vi "IZRCSM_ut_test_eng.vi"(8 "Error In":errorcluster, 11 "CSMinfo in":T2) -> (0 "Error Out":errorcluster, 3 "CSMinfo out":T2)   [LabVIEW 2018]
uses:
  IZRCSM.ctl
  IZRCSM_string2.ctl
  MOKO_LabViewLibrary/MokoSTM/MokoClassicUtilitySTM/MCUS_STM.ctl
  MOKO_LabViewLibrary/MokoSTM/MokoClassicUtilitySTM/MCUS_ITEM.ctl
panel:
  in  "Применить":bool
  in  "Температура окружающего воздуха":T1
  in  "Атмосферное давление":T1
  in  "Относительная влажность воздуха":T1
  # "0,4\n0,6\n1\n1,5\n1,6\n2,5\n4"
  # "kPa\nbar\nkgf/cm2\nMPa"
  # "Climatic conditions"
  # "Permissible range"
  # "Measured values"
  # "Measured parameter"
  # "Ambient temperature:"
  # "from +15,0 °C to +35,0 °C"
  # "Relative humidity:"
  # "from 45% to 80%"
  # "Atmosphere pressure:"
  # "from 84,0 to 106,7 kPa"
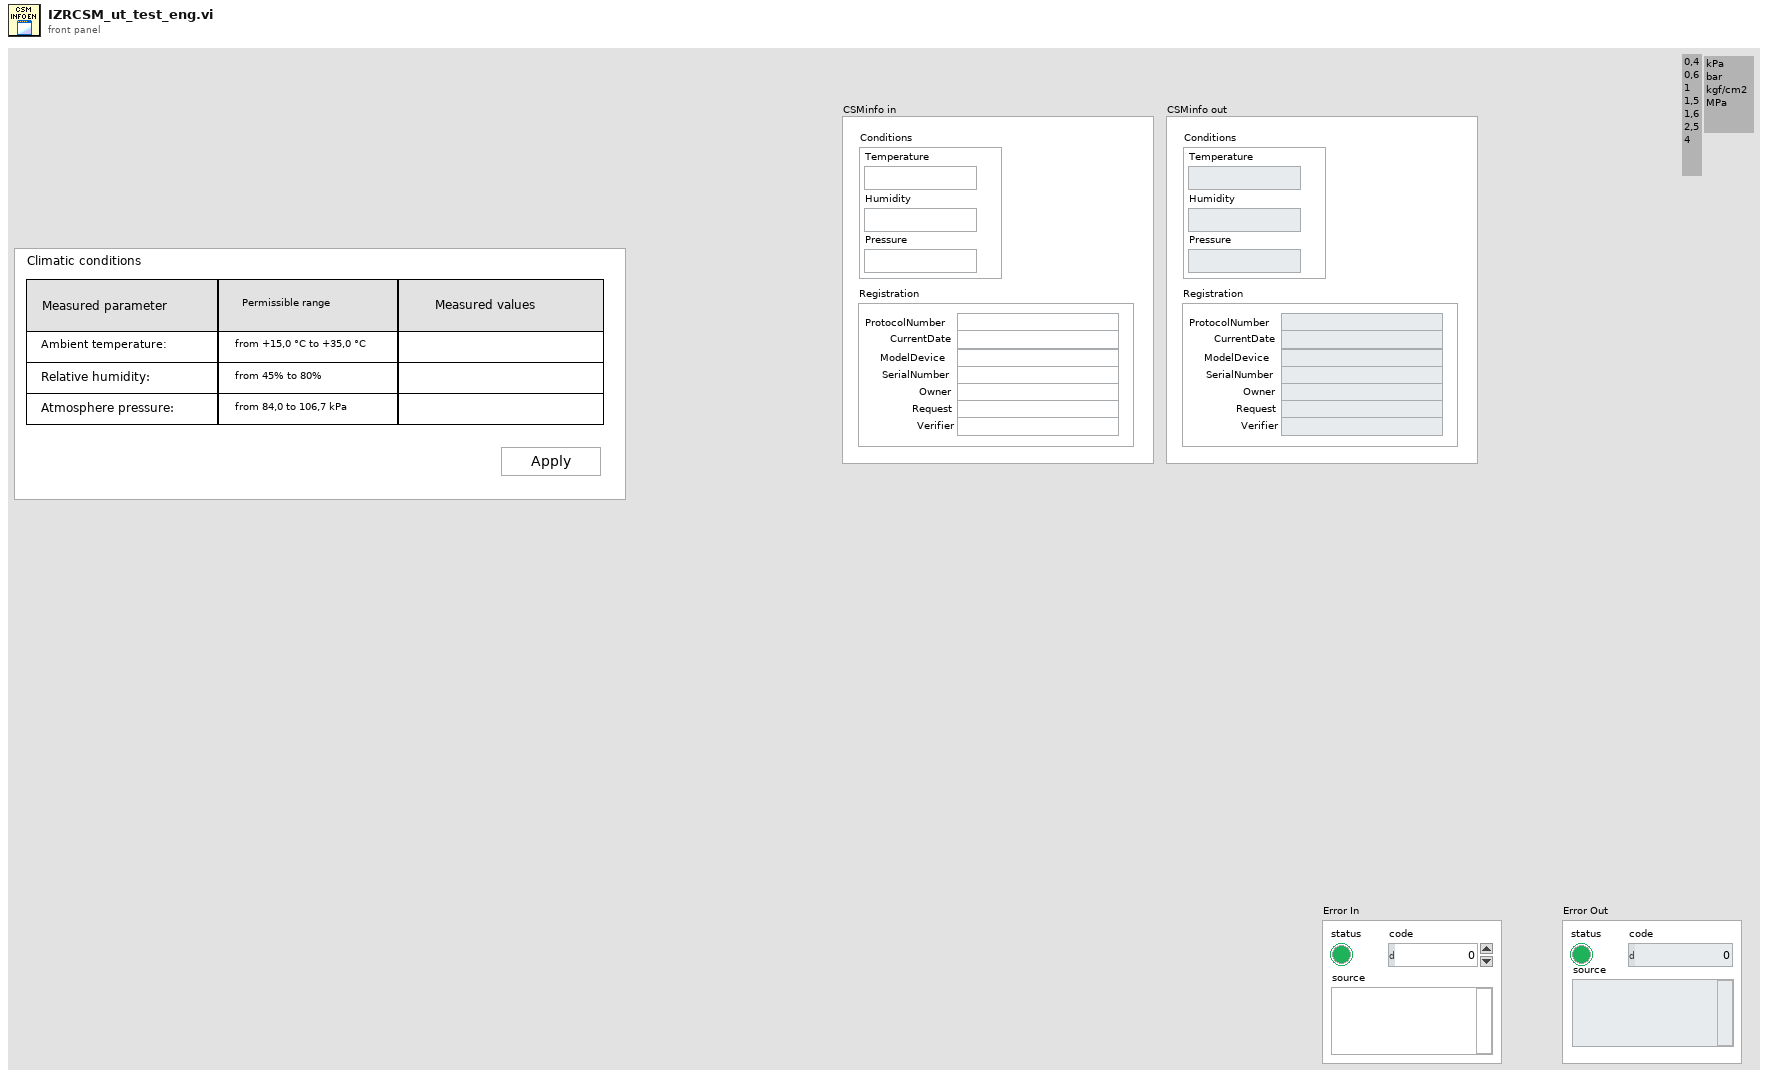
[diagram p1: front panel]
types:
  T1 = typedef "IZRCSM_string2.ctl" = string
  T2 = typedef "IZRCSM.ctl" = cluster{"Conditions":cluster{"Temperature":string, "Humidity":string, "Pressure":string}, "Registration":cluster{"ProtocolNumber":string, "CurrentDate":string, "ModelDevice":string, "SerialNumber":string, "Owner":string, "Request":string, "Verifier":string}}
  T3 = typedef "MCUS_STM.ctl" = cluster{"main stm":T4, "data":string}
  T4 = typedef "MCUS_ITEM.ctl" = enum16{"idle", "_____ main_____ ", "Init", "Stop", "Apply values", "Save", "Open", "Reset"}
  T5 = typedef "CSMinfo_string2.ctl" = string
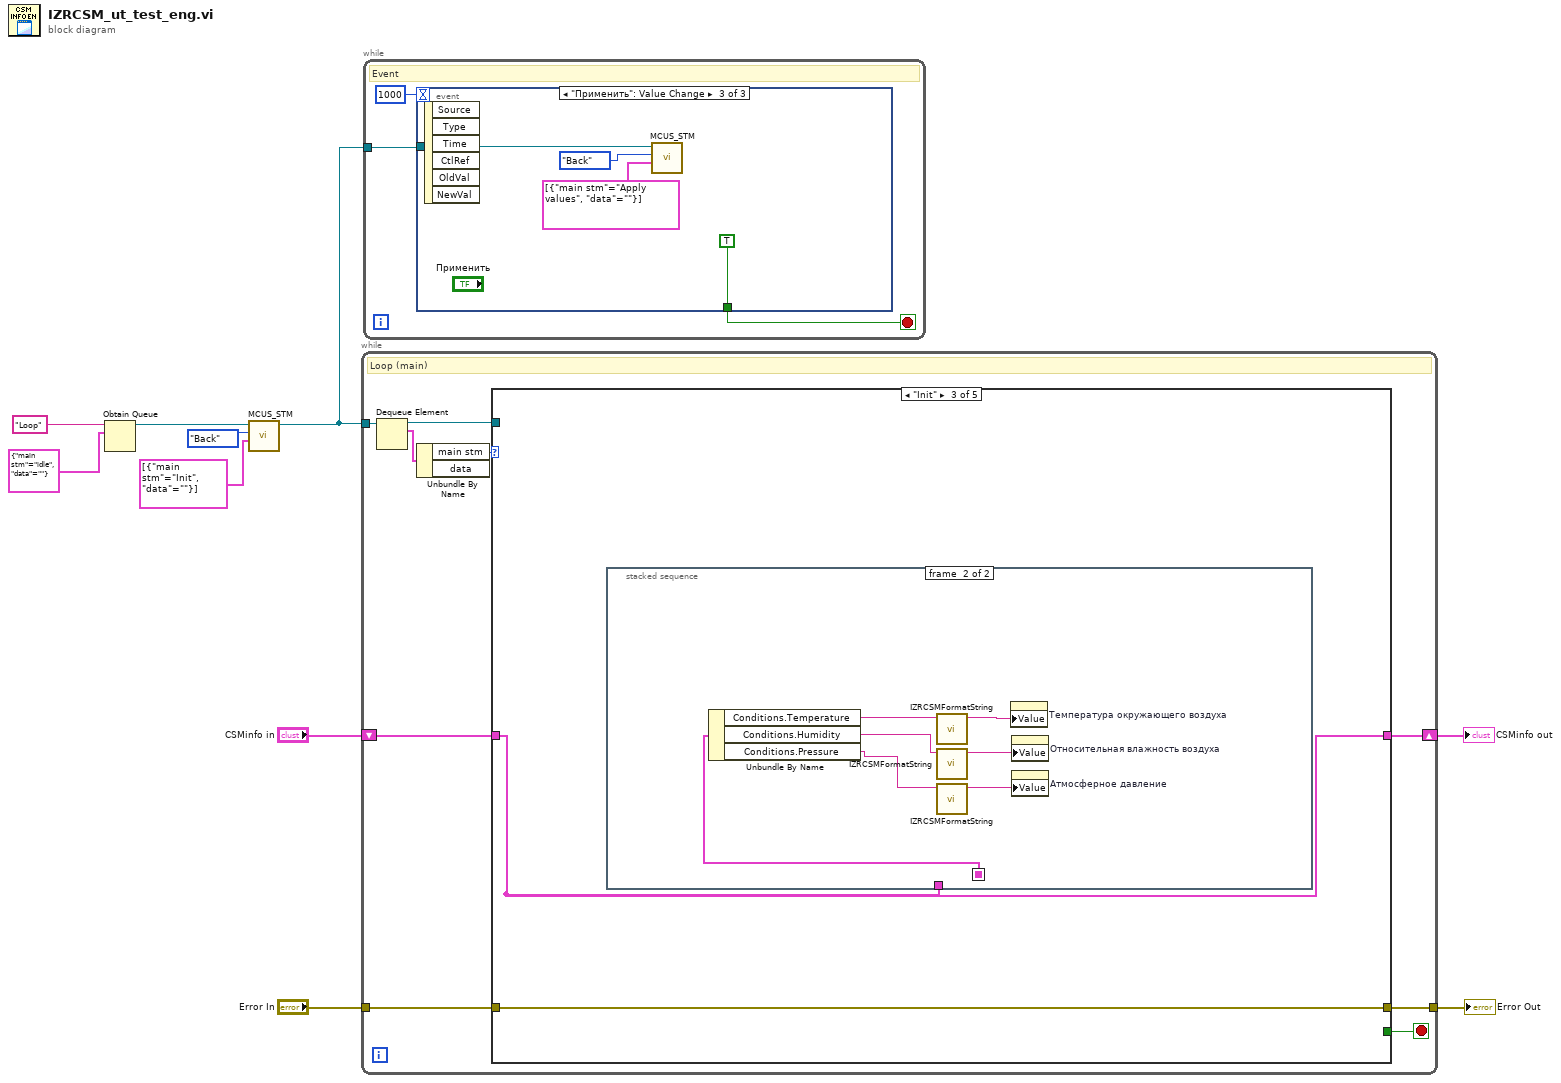
[diagram p0: block diagram]
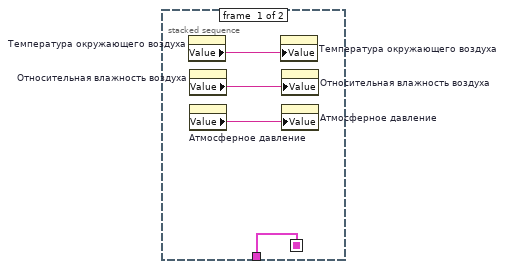
[diagram p4: hidden frame]
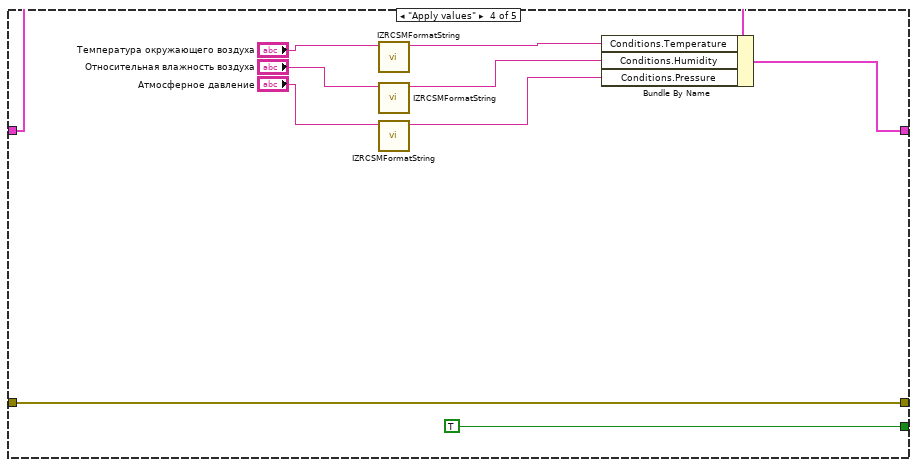
[diagram p5: hidden frame]
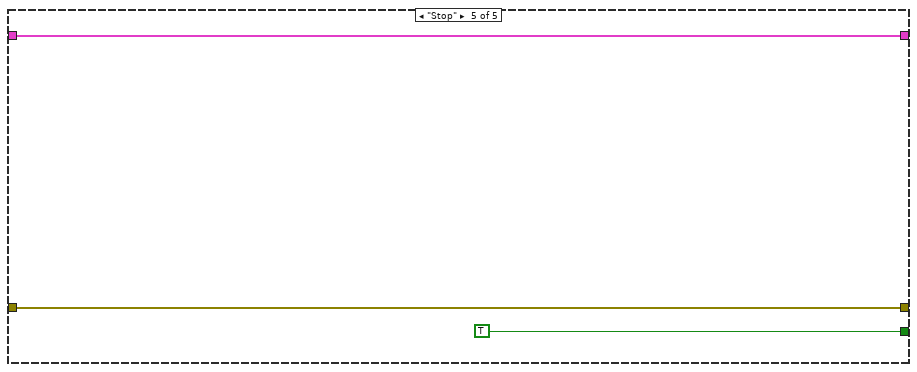
[diagram p6: hidden frame]
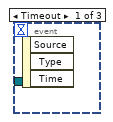
[diagram p7: hidden frame]
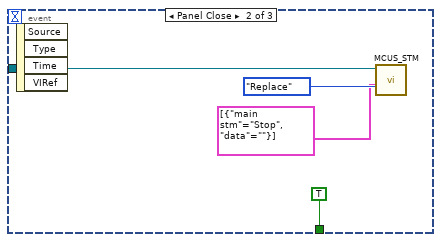
[diagram p8: hidden frame]
diagram:
  n1 = Obtain Queue(name (unnamed)="Loop", element data type=T3 {"main stm"=enum."idle", "data"=""} ("MOKO_NMEA")) -> (queue out=w10:refnum<queue>)  [unwired: 3 in, 2 out]
  n2 = call "MCUS_STM.vi"("StateMachineSteps"=T3[] [{"main stm"=enum."Init", "data"=""}], "FNs"=enum16{"Back", "Front", "Replace"}."Back", "Queue in"=w10) -> ("Queue out"=w5:refnum<queue>)  [unwired: 7 in, 1 out]
  n3 = while {
    tunnel: w5 -> [w19]
    tunnel: "Error In" -> [w12]
    tunnel: [w11] -> w1
    shift-right: [w14] -> w4
    shift-left: "CSMinfo in" -> [w13]
    stop <- w15 stop-if-true
    # "Loop (main)"
    n4 = Dequeue Element(queue=w19) -> (queue out=w18:refnum<queue>, element=w17:T3)  [unwired: 2 in, 2 out]
    n5 = Unbundle By Name(w17) -> ("main stm"=w16:T4)  [unwired: 1 out]
    n6 = case shown="\"Init\"" w16 {
      tunnel: w18 -> [_ _ _ _ _]
      tunnel: [_ _ _ TRUE TRUE] -> w15
      tunnel: [_ _ w20 w36 w44] -> w14
      tunnel: w13 -> [_ _ w20 w37 w44]
      tunnel: w12 -> [_ _ w21 w41 w43]
      tunnel: [_ _ w21 w41 w43] -> w11
      frame "idle", Default {
      }
      frame "_____ main_____ " {
      }
      frame "Init" {
        n7 = stacked-sequence {
          seq-local: [w25 _] -> [_ w26]
          tunnel: w20 -> [w25 _]
          frame #0 {
            n8 = property on="Температура окружающего воздуха" class="Str (strict)"() -> ("Value"=w24:T5)  [unwired: 2 in, 2 out]
            n9 = property on="Относительная влажность воздуха" class="Str (strict)"() -> ("Value"=w23:T5)  [unwired: 2 in, 2 out]
            n10 = property on="Атмосферное давление" class="Str (strict)"() -> ("Value"=w22:T5)  [unwired: 2 in, 2 out]
            n11 = property on="Температура окружающего воздуха" class="Str (strict)"("Value"=w24) -> ()  [unwired: 2 in, 2 out]
            n12 = property on="Относительная влажность воздуха" class="Str (strict)"("Value"=w23) -> ()  [unwired: 2 in, 2 out]
            n13 = property on="Атмосферное давление" class="Str (strict)"("Value"=w22) -> ()  [unwired: 2 in, 2 out]
          }
          frame #1 {
            n14 = Unbundle By Name(w26) -> ("Conditions.Temperature"=w29:string, "Conditions.Humidity"=w28:string, "Conditions.Pressure"=w27:string)
            n15 = call "IZRCSMFormatString.vi"("Input string"=w29) -> ("resulting string"=w31:string)  [unwired: 9 in, 1 out]
            n16 = call "IZRCSMFormatString.vi"("Input string"=w28) -> ("resulting string"=w30:string)  [unwired: 9 in, 1 out]
            n17 = call "IZRCSMFormatString.vi"("Input string"=w27) -> ("resulting string"=w32:string)  [unwired: 9 in, 1 out]
            n18 = property on="Температура окружающего воздуха" class="Str (strict)"("Value"=w31) -> ()  [unwired: 2 in, 2 out]
            n19 = property on="Относительная влажность воздуха" class="Str (strict)"("Value"=w30) -> ()  [unwired: 2 in, 2 out]
            n20 = property on="Атмосферное давление" class="Str (strict)"("Value"=w32) -> ()  [unwired: 2 in, 2 out]
          }
        }
      }
      frame "Apply values" {
        n21 = call "IZRCSMFormatString.vi"("Input string"="Температура окружающего воздуха") -> ("resulting string"=w35:string)  [unwired: 9 in, 1 out]
        n22 = call "IZRCSMFormatString.vi"("Input string"="Относительная влажность воздуха") -> ("resulting string"=w34:string)  [unwired: 9 in, 1 out]
        n23 = call "IZRCSMFormatString.vi"("Input string"="Атмосферное давление") -> ("resulting string"=w33:string)  [unwired: 9 in, 1 out]
        n24 = Bundle By Name(cluster=w37, "Conditions.Temperature"=w35, "Conditions.Humidity"=w34, "Conditions.Pressure"=w33) -> (w36:T2)
      }
      frame "Stop" {
      }
    }
  }
  "CSMinfo out" <- w4
  "Error Out" <- w1
  n25 = while {
    tunnel: w5 -> [w46]
    stop <- w48 stop-if-true
    # "Event"
    n26 = event shown="[2] \"Применить\": Value Change" {
      selector: _ -> [_ _ _]
      dyn-events: _ -> [_ _ _]
      timeout: 1000 -> [_ _ _]
      tunnel: [_ TRUE TRUE] -> w48
      tunnel: w46 -> [_ w49 w54]
      event Timeout {
        n27 = event-data() -> ()  [unwired: 1 in, 3 out]
      }
      event Panel Close {
        n28 = event-data() -> ()  [unwired: 1 in, 4 out]
        n29 = call "MCUS_STM.vi"("StateMachineSteps"=T3[] [{"main stm"=enum."Stop", "data"=""}], "FNs"=enum16{"Back", "Front", "Replace"}."Replace", "Queue in"=w49) -> ()  [unwired: 7 in, 2 out]
      }
      event "Применить": Value Change {
        n30 = event-data() -> ()  [unwired: 1 in, 6 out]
        n31 = call "MCUS_STM.vi"("StateMachineSteps"=T3[] [{"main stm"=enum."Apply values", "data"=""}], "FNs"=enum16{"Back", "Front", "Replace"}."Back", "Queue in"=w54) -> ()  [unwired: 7 in, 2 out]
      }
    }
  }
